vi "HW_Configure_port(s).vi"(0 "Settings cluster in":T2={"Defaults"={"Default User"=0.0, "VISA Resource Name "="", "Histogram parameters"={"max"=300.0, "min"=0.0, "# bins"=10, "threshold"=8.0, "thr. type"=enum."higher accepted"}}, "Recording and saving"={"Researcher name"="", "Name prefix"="", "Data post-processing"={"Filter type"=enum."Savitzky-Golay", "Length"=31, "Order"=3}, "Stop at"=0.0, "\"Stop at\" enabled"=FALSE, "Default save folder path"=path "", "Acquisition FPS"=enum."Max"}, "Geometry"={"Sensor board size"=enum."", "Bridge swap"=FALSE, "Twisted neck"=FALSE, "Bridge H. offset"=0.0, "Bridge V. offset"=0.0, "Magnets orientation"=0.0, "Cage type"=0, "Cage parameters"={"Round"=variant(i16 0), "Square"=variant(u16 0), "Donut-maze"=variant(u16 0), "T-maze"=variant(u8 0), "Sociability-maze"=variant(u8 0)}}, "IO parameters"={"IO general config."=0, "IO 1 configuration"=0, "IO 2 configuration"=0, "IO 3 configuration"=0, "IO 4 configuration"=0, "Activate ext. RS-232"=0, "IO inversion config."=0, "Sync capability"=1}, "Conditions presets array"=[{"Enabled"=FALSE, "Name"="", "Specifier(s)"=[], "Response"={"Response type"=enum."Air puff", "TTL port"=enum."Port 1", "TTL pulse length, ms"=0.0}, "Has been set"=FALSE}, {"Enabled"=FALSE, "Name"="", "Specifier(s)"=[], "Response"={"Response type"=enum."Air puff", "TTL port"=enum."Port 1", "TTL pulse length, ms"=0.0}, "Has been set"=FALSE}, {"Enabled"=FALSE, "Name"="", "Specifier(s)"=[], "Response"={"Response type"=enum."Air puff", "TTL port"=enum."Port 1", "TTL pulse length, ms"=0.0}, "Has been set"=FALSE}, {"Enabled"=FALSE, "Name"="", "Specifier(s)"=[], "Response"={"Response type"=enum."Air puff", "TTL port"=enum."Port 1", "TTL pulse length, ms"=0.0}, "Has been set"=FALSE}, {"Enabled"=FALSE, "Name"="", "Specifier(s)"=[], "Response"={"Response type"=enum."Air puff", "TTL port"=enum."Port 1", "TTL pulse length, ms"=0.0}, "Has been set"=FALSE}, {"Enabled"=FALSE, "Name"="", "Specifier(s)"=[], "Response"={"Response type"=enum."Air puff", "TTL port"=enum."Port 1", "TTL pulse length, ms"=0.0}, "Has been set"=FALSE}, {"Enabled"=FALSE, "Name"="", "Specifier(s)"=[], "Response"={"Response type"=enum."Air puff", "TTL port"=enum."Port 1", "TTL pulse length, ms"=0.0}, "Has been set"=FALSE}, {"Enabled"=FALSE, "Name"="", "Specifier(s)"=[], "Response"={"Response type"=enum."Air puff", "TTL port"=enum."Port 1", "TTL pulse length, ms"=0.0}, "Has been set"=FALSE}, {"Enabled"=FALSE, "Name"="", "Specifier(s)"=[], "Response"={"Response type"=enum."Air puff", "TTL port"=enum."Port 1", "TTL pulse length, ms"=0.0}, "Has been set"=FALSE}, {"Enabled"=FALSE, "Name"="", "Specifier(s)"=[], "Response"={"Response type"=enum."Air puff", "TTL port"=enum."Port 1", "TTL pulse length, ms"=0.0}, "Has been set"=FALSE}, {"Enabled"=FALSE, "Name"="", "Specifier(s)"=[], "Response"={"Response type"=enum."Air puff", "TTL port"=enum."Port 1", "TTL pulse length, ms"=0.0}, "Has been set"=FALSE}, {"Enabled"=FALSE, "Name"="", "Specifier(s)"=[], "Response"={"Response type"=enum."Air puff", "TTL port"=enum."Port 1", "TTL pulse length, ms"=0.0}, "Has been set"=FALSE}, {"Enabled"=FALSE, "Name"="", "Specifier(s)"=[], "Response"={"Response type"=enum."Air puff", "TTL port"=enum."Port 1", "TTL pulse length, ms"=0.0}, "Has been set"=FALSE}, {"Enabled"=FALSE, "Name"="", "Specifier(s)"=[], "Response"={"Response type"=enum."Air puff", "TTL port"=enum."Port 1", "TTL pulse length, ms"=0.0}, "Has been set"=FALSE}], "Calibration parameters"={"Timing calibration sw/hw"=1.0, "True FPS"=80.0, "True frame time, s"=80.0, "Disp. calibration info"=[]}, "Settings loaded OK"=FALSE} {"Calibration parameters"."True frame time, s" format="%.10g"; "Calibration parameters"."Disp. calibration info"."Speed, µl per ms" format="%.3g"; "Calibration parameters"."True FPS" format="%.10g"; "Calibration parameters"."Timing calibration sw/hw" format="%.10g"; "Conditions presets array"."Specifier(s)"."Validity criteria(s)"."Validity value" min=0.0 step=0.1 format="%.2g"; "Conditions presets array"."Specifier(s)"."Value" step=1.0 format="%#.2g"; "Recording and saving"."Data post-processing"."Order" min=3 max=11 step=2; "Recording and saving"."Data post-processing"."Length" min=5 max=301 step=2; "Geometry"."Cage type" items=["Round", "Square", "Donut-maze", "T-maze", "Sociability maze", ""]}, 1 "error in (no error)":errorcluster) -> (2 "Settings cluster out":T2={"Defaults"={"Default User"=0.0, "VISA Resource Name "="", "Histogram parameters"={"max"=300.0, "min"=0.0, "# bins"=10, "threshold"=8.0, "thr. type"=enum."higher accepted"}}, "Recording and saving"={"Researcher name"="", "Name prefix"="", "Data post-processing"={"Filter type"=enum."Savitzky-Golay", "Length"=31, "Order"=3}, "Stop at"=0.0, "\"Stop at\" enabled"=FALSE, "Default save folder path"=path "", "Acquisition FPS"=enum."Max"}, "Geometry"={"Sensor board size"=enum."", "Bridge swap"=FALSE, "Twisted neck"=FALSE, "Bridge H. offset"=0.0, "Bridge V. offset"=0.0, "Magnets orientation"=0.0, "Cage type"=0, "Cage parameters"={"Round"=variant(i16 0), "Square"=variant(u16 0), "Donut-maze"=variant(u16 0), "T-maze"=variant(u8 0), "Sociability-maze"=variant(u8 0)}}, "IO parameters"={"IO general config."=0, "IO 1 configuration"=0, "IO 2 configuration"=0, "IO 3 configuration"=0, "IO 4 configuration"=0, "Activate ext. RS-232"=0, "IO inversion config."=0, "Sync capability"=1}, "Conditions presets array"=[{"Enabled"=FALSE, "Name"="", "Specifier(s)"=[], "Response"={"Response type"=enum."Air puff", "TTL port"=enum."Port 1", "TTL pulse length, ms"=0.0}, "Has been set"=FALSE}, {"Enabled"=FALSE, "Name"="", "Specifier(s)"=[], "Response"={"Response type"=enum."Air puff", "TTL port"=enum."Port 1", "TTL pulse length, ms"=0.0}, "Has been set"=FALSE}, {"Enabled"=FALSE, "Name"="", "Specifier(s)"=[], "Response"={"Response type"=enum."Air puff", "TTL port"=enum."Port 1", "TTL pulse length, ms"=0.0}, "Has been set"=FALSE}, {"Enabled"=FALSE, "Name"="", "Specifier(s)"=[], "Response"={"Response type"=enum."Air puff", "TTL port"=enum."Port 1", "TTL pulse length, ms"=0.0}, "Has been set"=FALSE}, {"Enabled"=FALSE, "Name"="", "Specifier(s)"=[], "Response"={"Response type"=enum."Air puff", "TTL port"=enum."Port 1", "TTL pulse length, ms"=0.0}, "Has been set"=FALSE}, {"Enabled"=FALSE, "Name"="", "Specifier(s)"=[], "Response"={"Response type"=enum."Air puff", "TTL port"=enum."Port 1", "TTL pulse length, ms"=0.0}, "Has been set"=FALSE}, {"Enabled"=FALSE, "Name"="", "Specifier(s)"=[], "Response"={"Response type"=enum."Air puff", "TTL port"=enum."Port 1", "TTL pulse length, ms"=0.0}, "Has been set"=FALSE}, {"Enabled"=FALSE, "Name"="", "Specifier(s)"=[], "Response"={"Response type"=enum."Air puff", "TTL port"=enum."Port 1", "TTL pulse length, ms"=0.0}, "Has been set"=FALSE}, {"Enabled"=FALSE, "Name"="", "Specifier(s)"=[], "Response"={"Response type"=enum."Air puff", "TTL port"=enum."Port 1", "TTL pulse length, ms"=0.0}, "Has been set"=FALSE}, {"Enabled"=FALSE, "Name"="", "Specifier(s)"=[], "Response"={"Response type"=enum."Air puff", "TTL port"=enum."Port 1", "TTL pulse length, ms"=0.0}, "Has been set"=FALSE}, {"Enabled"=FALSE, "Name"="", "Specifier(s)"=[], "Response"={"Response type"=enum."Air puff", "TTL port"=enum."Port 1", "TTL pulse length, ms"=0.0}, "Has been set"=FALSE}, {"Enabled"=FALSE, "Name"="", "Specifier(s)"=[], "Response"={"Response type"=enum."Air puff", "TTL port"=enum."Port 1", "TTL pulse length, ms"=0.0}, "Has been set"=FALSE}, {"Enabled"=FALSE, "Name"="", "Specifier(s)"=[], "Response"={"Response type"=enum."Air puff", "TTL port"=enum."Port 1", "TTL pulse length, ms"=0.0}, "Has been set"=FALSE}, {"Enabled"=FALSE, "Name"="", "Specifier(s)"=[], "Response"={"Response type"=enum."Air puff", "TTL port"=enum."Port 1", "TTL pulse length, ms"=0.0}, "Has been set"=FALSE}], "Calibration parameters"={"Timing calibration sw/hw"=1.0, "True FPS"=80.0, "True frame time, s"=80.0, "Disp. calibration info"=[]}, "Settings loaded OK"=FALSE} {"Calibration parameters"."True frame time, s" format="%.10g"; "Calibration parameters"."Disp. calibration info"."Speed, µl per ms" format="%.3g"; "Calibration parameters"."True FPS" format="%.10g"; "Calibration parameters"."Timing calibration sw/hw" format="%.10g"; "Conditions presets array"."Specifier(s)"."Validity criteria(s)"."Validity value" min=0.0 step=0.1 format="%.2g"; "Conditions presets array"."Specifier(s)"."Value" step=1.0 format="%#.2g"; "Recording and saving"."Data post-processing"."Order" min=3 max=11 step=2; "Recording and saving"."Data post-processing"."Length" min=5 max=301 step=2; "Geometry"."Cage type" items=["Round", "Square", "Donut-maze", "T-maze", "Sociability maze", ""]}, 3 "Data updated":bool, 4 "error out":errorcluster)   [LabVIEW 2018, in "Common_Resources.lvlib"]
uses:
  Common_Resources.lvlib
  SubVi's/Controls/CTL_Undo_button.ctl
  SubVi's/Controls/CTL_Settings_cluster.ctl
  SubVi's/Controls/CTL_Histogram_parameters.ctl
  SubVi's/Controls/CTL_Filter_selector.ctl
  SubVi's/Controls/CTL_Acquisition_speed_selector.ctl
  Typedefs/CTL_Segmented_plot_parameters_2.ctl
  Libraries/Cage Diagram/Typedefs/CTL_Cage_type.ctl
  SubVi's/Controls/CTL_Cage_all_segmentation_params_set.ctl
  SubVi's/Controls/CTL_IO_params_cluster.ctl
  SubVi's/Controls/CTL_Conditions_Array.ctl
  SubVi's/Controls/CTL_Conditions_Cluster.ctl
  SubVi's/Controls/CTL_Condition_type.ctl
  SubVi's/Controls/CTL_Comparison_type.ctl
  SubVi's/Controls/CTL_Validity_check_criteria.ctl
  SubVi's/Controls/CTL_Response_info.ctl
  SubVi's/Controls/CTL_Condition_response_type.ctl
  SubVi's/Controls/CTL_Reponse_port_info.ctl
  SubVi's/Controls/CTL_Calibration_parameters.ctl
  SubVi's/Controls/CTL_Dispenser_calibration_info.ctl
  SubVi's/Controls/CTL_VISA_port_Descr.-Name.ctl
  <vilib>/Utility/miscctls.llb/LVPointTypeDef.ctl
  Libraries/Cage Diagram/Cage Diagram.lvlib
panel:
  out "Current port":string
  in  "COM-ports":i32(listbox)
  out "Detected COM ports":T1[](array[typedef])
  out "Previous parameters":cluster{"VISA resourse name":string}
  in  "Check HW":bool
  in  "Undo":T20
  in  "Save Config":bool
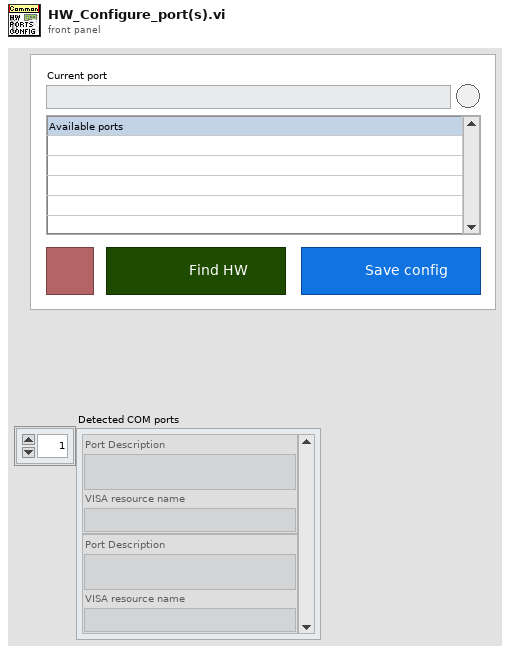
[diagram p1: front panel]
types:
  T1 = typedef "Common_Resources.lvlib/CTL_VISA_port_Descr.-Name.ctl" = cluster{"Port Description":string, "VISA resource name":string}
  T2 = typedef "Common_Resources.lvlib/CTL_Settings_cluster.ctl" = cluster{"Defaults":cluster{"Default User":dbl, "VISA Resource Name ":string, "Histogram parameters":T3}, "Recording and saving":cluster{"Researcher name":string, "Name prefix":string, "Data post-processing":T4, "Stop at":dbl, "\"Stop at\" enabled":bool, "Default save folder path":path, "Acquisition FPS":T5}, "Geometry":T6, "IO parameters":T9, "Conditions presets array":T10, "Calibration parameters":T18, "Settings loaded OK":bool}
  T3 = typedef "Common_Resources.lvlib/CTL_Histogram_parameters.ctl" = cluster{"max":dbl, "min":dbl, "# bins":i32, "threshold":dbl, "thr. type":enum16{"higher accepted", "lower accepted"}}
  T4 = typedef "Common_Resources.lvlib/CTL_Filter_selector.ctl" = cluster{"Filter type":enum16{"None", "Savitzky-Golay"}, "Length":i32, "Order":i32}
  T5 = typedef "Common_Resources.lvlib/CTL_Acquisition_speed_selector.ctl" = enum16{"Max", "Optimal", "Eco"}
  T6 = typedef "Common_Resources.lvlib/CTL_Segmented_plot_parameters_2.ctl" = cluster{"Sensor board size":enum16{"", "Large"}, "Bridge swap":bool, "Twisted neck":bool, "Bridge H. offset":sgl, "Bridge V. offset":sgl, "Magnets orientation":sgl, "Cage type":T7, "Cage parameters":T8}
  T7 = typedef "Cage Diagram.lvlib/CTL_Cage_type.ctl" = u16
  T8 = typedef "Common_Resources.lvlib/CTL_Cage_all_segmentation_params_set.ctl" = cluster{"Round":variant, "Square":variant, "Donut-maze":variant, "T-maze":variant, "Sociability-maze":variant}
  T9 = typedef "Common_Resources.lvlib/CTL_IO_params_cluster.ctl" = cluster{"IO general config.":u16, "IO 1 configuration":u16, "IO 2 configuration":u16, "IO 3 configuration":u16, "IO 4 configuration":u16, "Activate ext. RS-232":u16, "IO inversion config.":u16, "Sync capability":u8}
  T10 = typedef "Common_Resources.lvlib/CTL_Conditions_Array.ctl" = T11[]
  T11 = typedef "Common_Resources.lvlib/CTL_Conditions_Cluster.ctl" = cluster{"Enabled":bool, "Name":string, "Specifier(s)":cluster{"Specifier enabled":bool, "Condition type":T12, "Comparison type":T13, "Value":dbl, "Validity criteria(s)":cluster{"V. check enabled":bool, "Criteria":T14, "Validity value":dbl}[]}[], "Response":T15, "Has been set":bool}
  T12 = typedef "Common_Resources.lvlib/CTL_Condition_type.ctl" = enum16{"Speed", "Zone", "Angle to wall"}
  T13 = typedef "Common_Resources.lvlib/CTL_Comparison_type.ctl" = enum16{"Less", "Less or Equal", "Equal", "Greater or Equal", "Greater", "Not Equal"}
  T14 = typedef "Common_Resources.lvlib/CTL_Validity_check_criteria.ctl" = enum16{"Running bout (seconds)", "Running bout (meters)"}
  T15 = typedef "Common_Resources.lvlib/CTL_Response_info.ctl" = cluster{"Response type":T16, "TTL port":T17, "TTL pulse length, ms":dbl}
  T16 = typedef "Common_Resources.lvlib/CTL_Condition_response_type.ctl" = enum16{"None", "Air puff", "Liquid reward", "TTL pulse", "TTL pulse (ubr)", "TTL signal"}
  T17 = typedef "Common_Resources.lvlib/CTL_Reponse_port_info.ctl" = enum16{"Port 1", "Port 2", "Port 3", "Port 4"}
  T18 = typedef "Common_Resources.lvlib/CTL_Calibration_parameters.ctl" = cluster{"Timing calibration sw/hw":dbl, "True FPS":dbl, "True frame time, s":dbl, "Disp. calibration info":T19}
  T19 = typedef "Common_Resources.lvlib/CTL_Dispenser_calibration_info.ctl" = cluster{"Channel":u8, "Speed, µl per ms":dbl}[]
  T20 = typedef "Common_Resources.lvlib/CTL_Undo_button.ctl" = bool
  T21 = typedef "LVPointTypeDef.ctl" = cluster{"Horizontal":i16, "Vertical":i16}
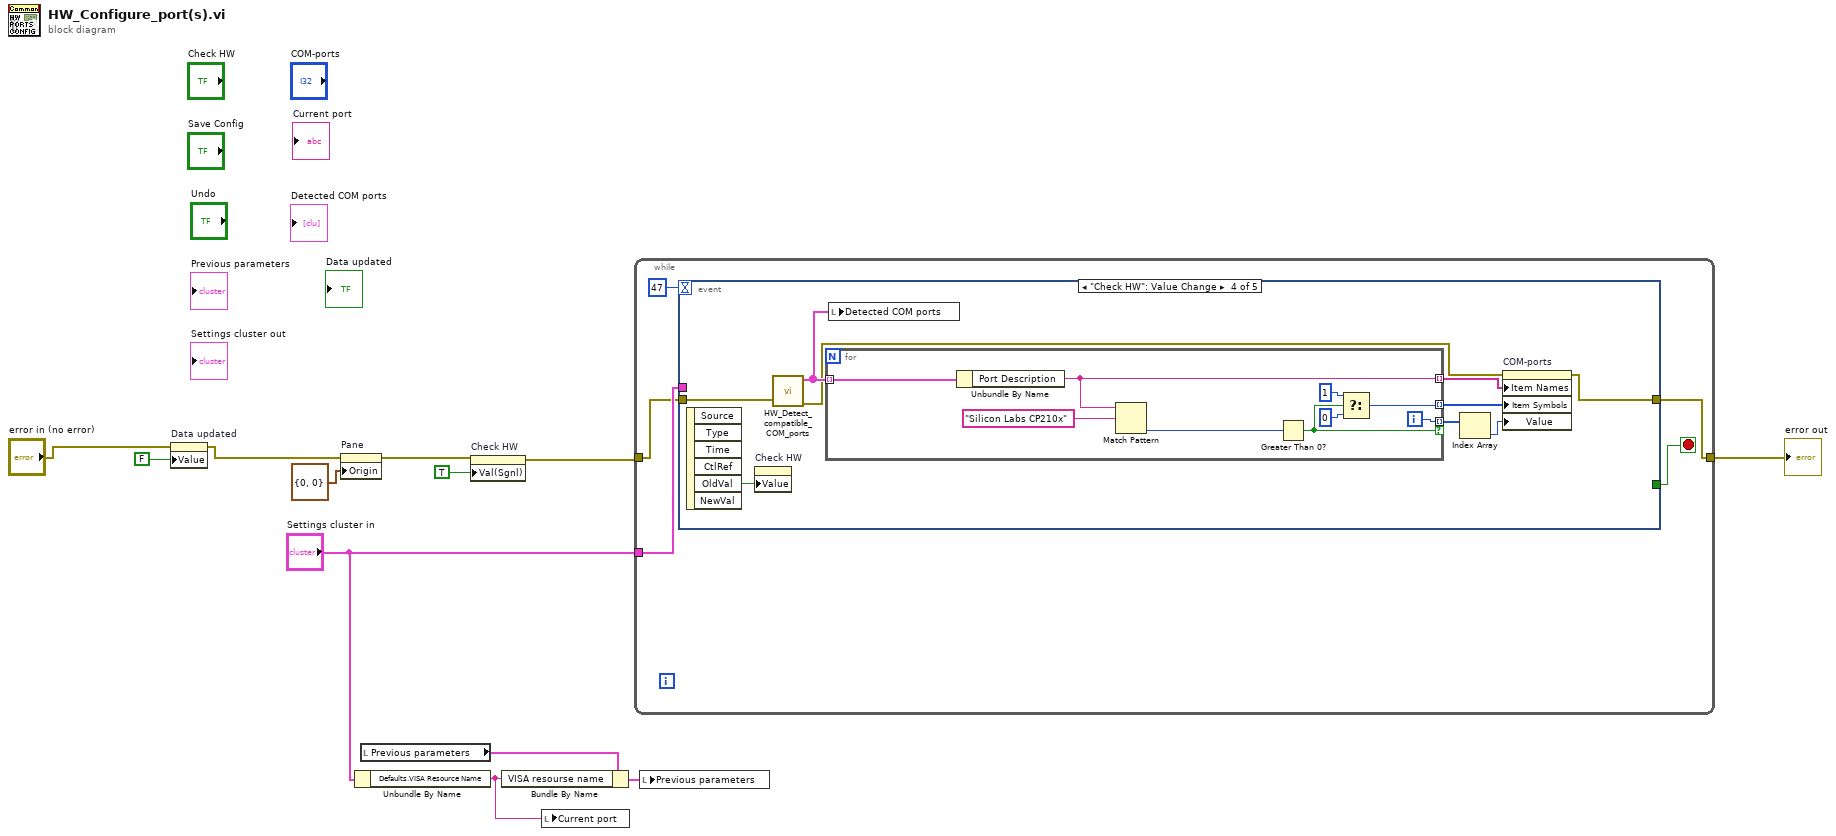
[diagram p0: block diagram]
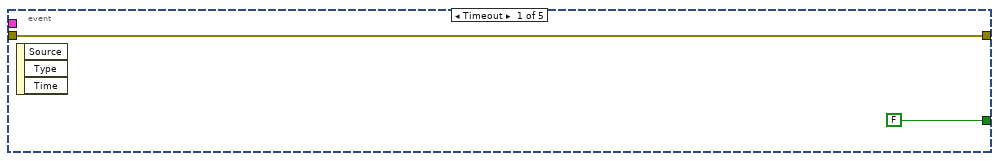
[diagram p2: hidden frame]
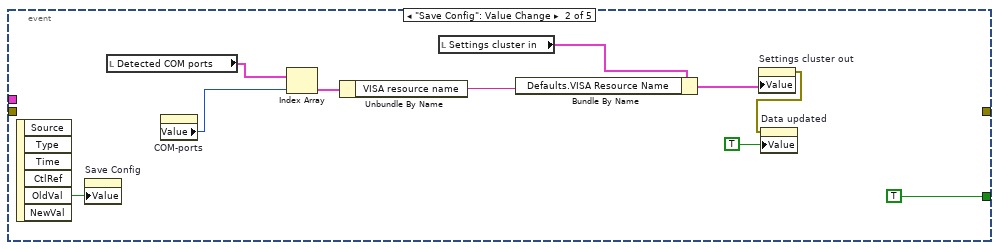
[diagram p3: hidden frame]
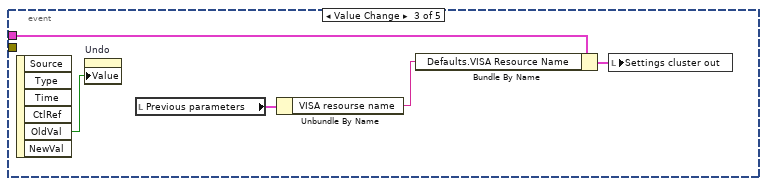
[diagram p4: hidden frame]
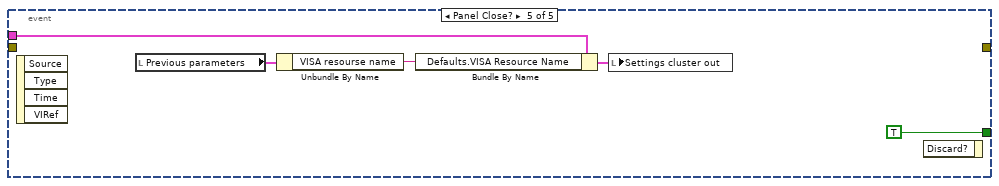
[diagram p5: hidden frame]
diagram:
  n1 = property on="Data updated" class="Bool (strict)"(error in="error in (no error)", "Value"=FALSE ("Data updated")) -> (error out=w2:errorcluster)  [unwired: 1 in, 1 out]
  n2 = property on="Pane" class="Pane"(error in=w2, "Origin"=T21 {"Horizontal"=0, "Vertical"=0}) -> (error out=w7:errorcluster)  [unwired: 1 in, 1 out]
  n3 = Unbundle By Name("Settings cluster in") -> ("Defaults.VISA Resource Name"=w4:string)
  n4 = local read "Previous parameters"() -> (w9:cluster{"VISA resourse name":string})
  n5 = property on="Check HW" class="Bool (strict)"(error in=w7, "Val(Sgnl)"=TRUE ("Value (Signaling)")) -> (error out=w6:errorcluster)  [unwired: 1 in, 1 out]
  n6 = Bundle By Name(cluster=w9, "VISA resourse name"=w4) -> (w8:cluster{"VISA resourse name":string})
  n7 = local write "Current port"(w4) -> ()
  n8 = while {
    tunnel: "Settings cluster in" -> [w15]
    tunnel: w6 -> [w13]
    tunnel: [w14] -> w11
    stop <- w16 stop-if-true
    n9 = event shown="[3] \"Check HW\": Value Change" {
      selector: _ -> [_ _ _ _ _]
      dyn-events: _ -> [_ _ _ _ _]
      timeout: 47 -> [_ _ _ _ _]
      tunnel: [FALSE TRUE _ _ TRUE] -> w16
      tunnel: w15 -> [_ _ w33 _ w56]
      tunnel: [w18 _ _ w36 _] -> w14
      tunnel: w13 -> [w18 _ _ w42 _]
      event Timeout {
        n10 = event-data() -> ()  [unwired: 1 in, 3 out]
      }
      event "Save Config": Value Change {
        n11 = event-data() -> ("OldVal"=w28:bool)  [unwired: 1 in, 5 out]
        n12 = property on="Save Config" class="Bool (strict)"("Value"=w28) -> ()  [unwired: 2 in, 2 out]
        n13 = local read "Detected COM ports"() -> (w27:T1[])
        n14 = property on="COM-ports" class="LstBox (strict)"() -> ("Value"=w26:i32)  [unwired: 2 in, 2 out]
        n15 = Index Array(array=w27, index=w26) -> (element=w25:T1)
        n16 = Unbundle By Name(w25) -> ("VISA resource name"=w24:string)
        n17 = local read "Settings cluster in"() -> (w20:T2)
        n18 = Bundle By Name(cluster=w20, "Defaults.VISA Resource Name"=w24) -> (w23:T2)
        n19 = property on="Settings cluster out" class="Clust (strict)"("Value"=w23) -> (error out=w21:errorcluster)  [unwired: 2 in, 1 out]
        n20 = property on="Data updated" class="Bool (strict)"(error in=w21, "Value"=TRUE ("Data updated")) -> ()  [unwired: 1 in, 2 out]
      }
      event Value Change {
        n21 = event-data() -> ("OldVal"=w34:T20)  [unwired: 1 in, 5 out]
        n22 = property on="Undo" class="Bool (strict)"("Value"=w34) -> ()  [unwired: 2 in, 2 out]
        n23 = local read "Previous parameters"() -> (w32:cluster{"VISA resourse name":string})
        n24 = Unbundle By Name(w32) -> ("VISA resourse name"=w31:string)
        n25 = Bundle By Name(cluster=w33, "Defaults.VISA Resource Name"=w31) -> (w30:T2)
        n26 = local write "Settings cluster out"(w30) -> ()
      }
      event "Check HW": Value Change {
        n27 = event-data() -> ("OldVal"=w43:bool)  [unwired: 1 in, 5 out]
        n28 = property on="Check HW" class="Bool (strict)"("Value"=w43) -> ()  [unwired: 2 in, 2 out]
        n29 = call "HW_Detect_compatible_COM_ports.vi"("Error In"=w42) -> ("Detected COM ports"=w37:T1[], "Error Out"=w35:errorcluster)  [unwired: 1 in, 2 out]
        n30 = for {
          tunnel: w37 -> [w52] mode=indexing
          tunnel: [w51] -> w41 mode=indexing
          tunnel: [w48] -> w39 mode=indexing if=w47
          tunnel: [w46] -> w40 mode=indexing
          i -> [w48]
          n31 = Unbundle By Name(w52) -> ("Port Description"=w51:string)
          n32 = Match Pattern(string=w51, regular expression="Silicon Labs CP210x") -> (offset past match=w49:i32)  [unwired: 1 in, 3 out]
          n33 = Greater Than 0?(x=w49) -> (x > 0?=w47:bool)
          n34 = Select(t=1, s=w47, f=0) -> (s? t:f=w46:i32)
        }
        n35 = local write "Detected COM ports"(w37) -> ()
        n36 = Index Array(array=w39) -> (element=w38:i32)  [unwired: 1 in]
        n37 = property on="COM-ports" class="LstBox (strict)"(error in=w35, "Item Names"=w41, "Item Symbols"=w40, "Value"=w38) -> (error out=w36:errorcluster)  [unwired: 1 in, 1 out]
      }
      event Panel Close? {
        n38 = event-data() -> ()  [unwired: 1 in, 4 out]
        n39 = local read "Previous parameters"() -> (w53:cluster{"VISA resourse name":string})
        n40 = Unbundle By Name(w53) -> ("VISA resourse name"=w55:string)
        n41 = Bundle By Name(cluster=w56, "Defaults.VISA Resource Name"=w55) -> (w54:T2)
        n42 = local write "Settings cluster out"(w54) -> ()
        n43 = event-data() -> ()  [unwired: 2 in, 1 out]
      }
    }
  }
  "error out" <- w11
  n44 = local write "Previous parameters"(w8) -> ()
